vi "FTW-Actor-Child-Remove.vi"(0 "FTW-ActorInstance In":refnum<class "FTW-ActorInstance.lvclass">, 5 "Connector Name":string, 11 "error in":errorcluster) -> (4 "FTW-ActorInstance Out":refnum<class "FTW-ActorInstance.lvclass">, 15 "error out":errorcluster)   [LabVIEW 2015, in "FTW-ActorInstance.lvclass"]
uses:
  FTW-ActorInstance.lvclass
  FTW-ActorInstance.lvclass/FTW-ActorInstance.ctl
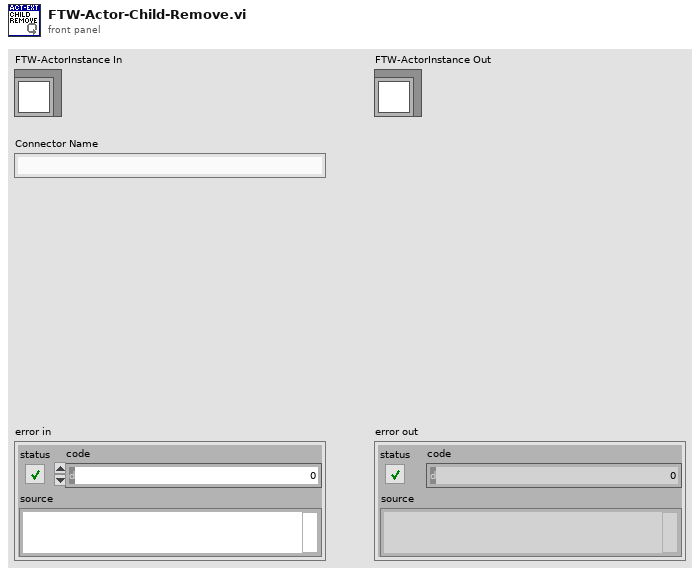
[diagram p1: front panel]
types:
  T1 = cluster{"Name":string, "URI":string, "Connector":refnum<class "FTW-ActorConnector.lvclass">, "Child":bool}[]
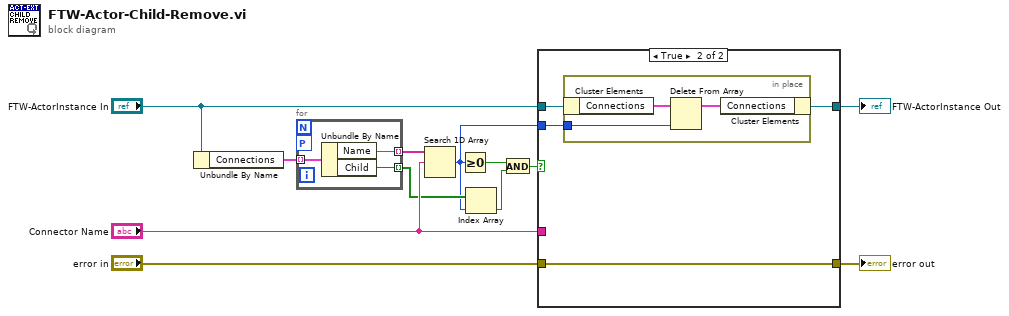
[diagram p0: block diagram]
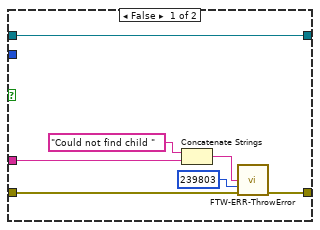
[diagram p2: hidden frame]
diagram:
  n1 = Unbundle By Name("FTW-ActorInstance In") -> ("Connections"=w12:T1)
  n2 = for {
    tunnel: w12 -> [w15] mode=indexing
    tunnel: [w14] -> w8 mode=indexing
    workers-P: _ -> [_]
    tunnel: [w13] -> w3 mode=indexing
    n3 = Unbundle By Name(w15) -> ("Name"=w14:string, "Child"=w13:bool)
  }
  n4 = Search 1D Array(1D array=w8, element="Connector Name") -> (index of element=w1:i32)  [unwired: 1 in]
  n5 = Greater Or Equal To 0?(x=w1) -> (x >= 0?=w5:bool)
  n6 = Index Array(array=w3, index=w1) -> (element=w2:bool)
  n7 = And(x=w5, y=w2) -> (x .and. y?=w4:bool)
  n8 = case shown="True" w4 {
    tunnel: [w21 w26] -> w11
    tunnel: "error in" -> [w22 w26]
    tunnel: "Connector Name" -> [w17 _]
    tunnel: [w16 w24] -> w7
    tunnel: "FTW-ActorInstance In" -> [w16 w25]
    tunnel: w1 -> [_ w23]
    frame False {
      n9 = Concatenate Strings("Could not find child " ("Error Message"), w17) -> (w18:string)
      n10 = call "FTW-ERR-ThrowError.vi"("Error Message"=w18, "Error Code"=239803, "error in"=w22) -> ("error out"=w21:errorcluster)  [unwired: 12 in]
    }
    frame True {
      n11 = in-place {
        in-place-border: w23 -> [w27]
        n12 = in-place-cluster #1(w25) -> ("Connections"=w28:T1)
        n13 = Delete From Array(array=w28, index=w27) -> (array with subset deleted=w29:T1)  [unwired: 1 in, 1 out]
        n14 = in-place-cluster #1("Connections"=w29) -> (w24:refnum<class "FTW-ActorInstance.lvclass">)
      }
    }
  }
  "FTW-ActorInstance Out" <- w7
  "error out" <- w11
